vi "GenerateMenuItems.vi"(8 "Bands":u16(ring) items=["No Bands", "A Octaves", "Curtin Bands", "JC violin 200-7000 Flat", "JC violin 200-780-1740-2930-7000", "JC violin 200-780-7000", "ObieAlto 200-650-1500-2700-6300"], 9 "View Type":u16(ring) items=["As measured"=0, "Normalize"=1, "Averaged"=3], 11 "Menu in":refnum<k9>) -> (0 "error out":errorcluster)   [LabVIEW 2022 SP3]
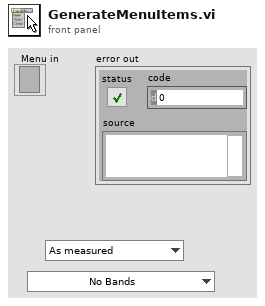
[diagram p1: front panel]
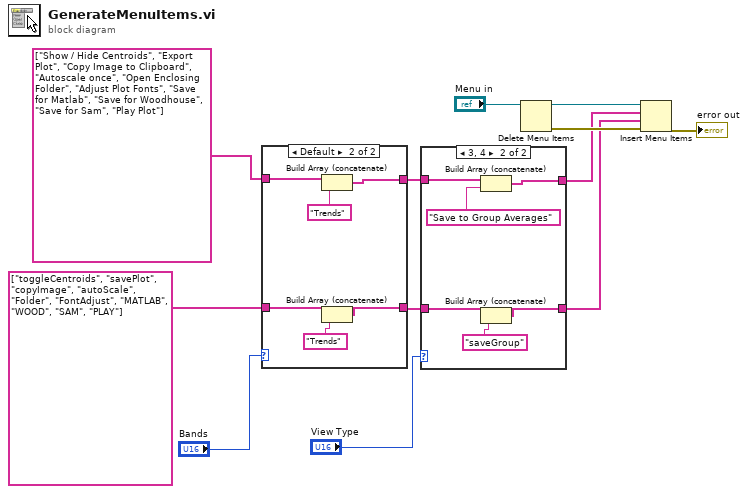
[diagram p0: block diagram]
diagram:
  n1 = case shown="Default" "Bands" {
    tunnel: string[] ["Show / Hide Centroids", "Export Plot", "Copy Image to Clipboard", "Autoscale once", "Open Enclosing Folder", "Adjust Plot Fonts", "Save for Matlab", "Save for Woodhouse", "Save for Sam", "Play Plot"] ("L10n_Parent Menus") -> [w14 w20]
    tunnel: [w14 w19] -> w4
    tunnel: string[] ["toggleCentroids", "savePlot", "copyImage", "autoScale", "Folder", "FontAdjust", "MATLAB", "WOOD", "SAM", "PLAY"] -> [w13 w18]
    tunnel: [w13 w17] -> w2
    frame 0 {
    }
    frame Default {
      n2 = Build Array (concatenate)(w20, "Trends" ("L10n_menu item")) -> (w19:string[])
      n3 = Build Array (concatenate)(w18, "Trends") -> (w17:string[])
    }
  }
  n4 = case shown="3, 4" "View Type" {
    tunnel: w4 -> [w22 w28]
    tunnel: [w22 w27] -> w7
    tunnel: w2 -> [w21 w26]
    tunnel: [w21 w25] -> w6
    frame Default {
    }
    frame 3, 4 {
      n5 = Build Array (concatenate)(w28, "Save to Group Averages" ("L10n_menu item")) -> (w27:string[])
      n6 = Build Array (concatenate)(w26, "saveGroup") -> (w25:string[])
    }
  }
  n7 = Delete Menu Items(9:"Menu in") -> (0:w10:errorcluster, 3:w9:refnum<k9>)  [unwired: 3 in]
  n8 = Insert Menu Items(6:w10, 7:w6, 8:w7, 9:w9) -> (0:→"error out":errorcluster)  [unwired: 2 in, 2 out]
